vi "ClearAll.vi"(8 "error in":errorcluster) -> (0 "error out":errorcluster)   [LabVIEW 2016]
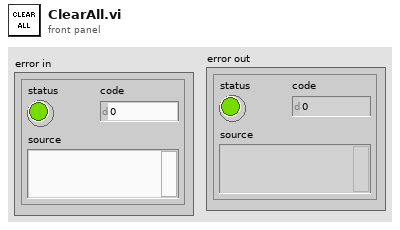
[diagram p1: front panel]
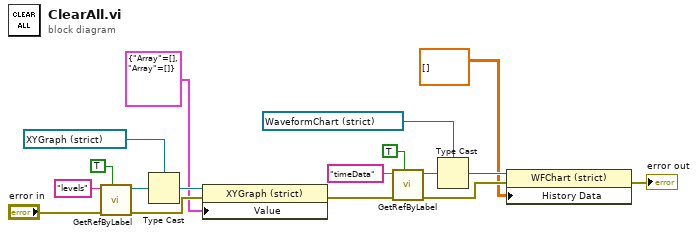
[diagram p0: block diagram]
diagram:
  n1 = call "GetRefByLabel.vi"("InsideTab"=TRUE, "error in"="error in", "Label"="levels") -> ("error out"=w13:errorcluster, "Ctl Refnum"=w15:refnum<vi>)  [unwired: 6 in, 1 out]
  n2 = Type Cast(type=refnum<vi> refnum ("levels"), x=w15) -> (*(type *) &x=w14:refnum<vi>)
  n3 = property class="XYGraph (strict)"(reference=w14, error in=w13, "Value"=cluster{"Array":i32[], "Array":dbl[]} {"Array"=[], "Array"=[]}) -> (error out=w10:errorcluster)  [unwired: 1 out]
  n4 = call "GetRefByLabel.vi"("InsideTab"=TRUE, "error in"=w10, "Label"="timeData") -> ("error out"=w8:errorcluster, "Ctl Refnum"=w7:refnum<vi>)  [unwired: 6 in, 1 out]
  n5 = Type Cast(type=refnum<vi> refnum ("timeData"), x=w7) -> (*(type *) &x=w6:refnum<vi>)
  n6 = property class="WFChart (strict)"(reference=w6, error in=w8, "History Data"=dbl[][] []) -> (error out=→"error out":errorcluster)  [unwired: 1 out]
